vi "XDCRDefaultReader.vi"(11 "path to XML document":path=path "C:/Labview Suite/ScanningControl/Location Specific/StonyBrook/DualXDCRSettings.xml") -> (0 "Dual XDCR Settings":T1 {"XDCR Settings"."UT340 Controls"."Low Pass Filter (MHz)" min=20 step=1; "XDCR Settings"."UT340 Controls"."High Pass Filter (MHz)" min=1 max=20 step=1; "XDCR Settings"."UT340 Controls"."Pulse Width (ns)" min=2.0 max=71.75; "XDCR Settings"."UT340 Controls"."Voltage" min=100 max=250 step=2; "XDCR Settings"."UT340 Controls"."PC Gain (dB)" min=-6 max=60 step=1; "XDCR Settings"."UT340 Controls"."PE Gain (dB)" min=-6 max=60 step=1; "XDCR Settings"."JSR Complete"."JSR Trigger Settings"."PRF (Hz)" items=["100 Hz"=0.1, "200 Hz"=0.2, "400 Hz"=0.4, "600 Hz"=0.6, "800 Hz"=0.8, "1000 Hz"=1.0, "1250 Hz"=1.25, "1500 Hz"=1.5, "1750 Hz"=1.75, "2000 Hz"=2.0, "2500 Hz"=2.5, "3000 Hz"=3.0, "3500 Hz"=3.5, "4000 Hz"=4.0, "4500 Hz"=4.5, "5000 Hz"=5.0]; "XDCR Settings"."JSR Complete"."JSR Trigger Settings"."Trigger Source" items=["Internal", "External"]; "XDCR Settings"."JSR Complete"."JSR Trigger Settings"."External Trigger Limit" items=["No Limit", "5 kHz"]; "XDCR Settings"."JSR Complete"."JSR Receive Settings"."Gain (dB)" min=-13 max=66 step=1; "XDCR Settings"."JSR Complete"."JSR Receive Settings"."Low Pass Filter" items=["5 MHz"=5, "10 MHz"=10, "15 MHz"=15, "22.5 MHz"=22, "35 MHz"=35, "50 MHz"=50]; "XDCR Settings"."JSR Complete"."JSR Receive Settings"."High Pass Filter" items=["DC"=0, "1 MHz"=1000, "2.5 MHz"=2500, "5 MHz"=5000, "7.5 MHz"=7500, "12.5 MHz"=12500]; "XDCR Settings"."JSR Complete"."JSR Receive Settings"."Receiver Mode" items=["Echo", "Through"]; "XDCR Settings"."JSR Complete"."JSR Pulse Settings"."Pulser Voltage (V)" items=["100"=100, "125"=125, "150"=150, "175"=175, "200"=200, "225"=225, "250"=250, "275"=275, "300"=300, "325"=325, "350"=350, "375"=375, "400"=400, "425"=425, "450"=450, "475"=475]; "XDCR Settings"."JSR Complete"."JSR Pulse Settings"."Pulser Impedance" items=["High z", "Low z"]; "XDCR Settings"."JSR Complete"."JSR Pulse Settings"."Pulse Energy Level" items=["0 (Minimum)", "1", "2", "3 (Maximum)"]; "XDCR Settings"."JSR Complete"."JSR Pulse Settings"."Damping" items=["331 Ohms"=331, "198 Ohms"=198, "142 Ohms"=142, "110 Ohms"=110, "92 Ohms"=92, "77 Ohms"=77, "67 Ohms"=67, "59 Ohms"=59, "52 Ohms"=52, "47 Ohms"=47, "43 Ohms"=43, "39 Ohms"=39, "37 Ohms"=37, "34 Ohms"=34, "32 Ohms"=32, "30 Ohms"=30]; "XDCR Settings"."Panametrics Settings"."FINE ATTENUATION" items=["00.0", "00.5", "01.0", "01.5", "02.0", "02.5", "03.0", "03.5", "04.0", "04.5", "05.0", "05.5", "06.0", "06.5", "07.0", "07.5", "08.0", "08.5", "09.0", "09.5", "10.0", "10.5", "11.0", "11.5", "12.0", "12.5", "13.0", "13.5", "14.0", "14.5", "15.0", "15.5"]; "XDCR Settings"."Panametrics Settings"."COARSE ATTENUATION" items=["00.0", "10.0", "20.0", "30.0", "40.0", "50.0"]; "XDCR Settings"."Panametrics Settings"."GAIN (db)" items=["26.0", "40.0", "54.0"]; "XDCR Settings"."Panametrics Settings"."PRF (KHz)" items=["XREMT", "EXBNC", "0.200", "0.500", "1.000", "2.000", "5.000", "10.00", "20.00"]; "XDCR Settings"."Panametrics Settings"."MODE" items=["P/ E", "THRU", "RPP", "EXT_PLSR"]; "XDCR Settings"."Panametrics Settings"."LP FILT (MHz)" items=["20", "50", "100", "200"]; "XDCR Settings"."Panametrics Settings"."HP FILT (KHz)" items=["1", "1000", "3000", "10000"]; "XDCR Settings"."Panametrics Settings"."DAMPING (Ohm)" items=["7", "10", "16", "20", "26", "30", "40", "50"]; "XDCR Settings"."Panametrics Settings"."ENERGY (uJ)" items=["1", "2", "4", "8", "16", "32"]; "XDCR Settings"."Daxsonics Settings"."Freq (MHz)" items=["4"=4, "5"=5, "6"=6, "8"=8, "10"=10, "12"=12, "14"=14, "15"=15, "16"=16, "17"=17, "18"=18, "20"=20, "25"=25, "30"=30, "35"=35, "40"=40, "45"=45, "50"=50]; "XDCR Settings"."Daxsonics Settings"."Voltage (V)" items=["0"=0, "5"=5, "10"=10, "15"=15, "20"=20, "25"=25, "30"=30, "35"=35, "40"=40, "45"=45, "50"=50, "55"=55, "60"=60, "65"=65, "70"=70, "75"=75, "80"=80, "85"=85, "90"=90, "95"=95, "100"=100, "110"=110, "120"=120, "130"=130, "140"=140, "150"=150, "160"=160, "170"=170, "180"=180, "190"=190]; "XDCR Settings"."Daxsonics Settings"."Gain (dB)" items=["22"=22, "25"=25, "28"=28, "31"=31, "34"=34, "37"=37, "40"=40, "43"=43, "46"=46, "49"=49, "52"=52, "55"=55, "58"=58, "61"=61, "64"=64, "67"=67]; "XDCR Settings"."Digitizer Settings"."Additional dig delay (ms)" format="%.2f"; "XDCR Settings"."Digitizer Settings"."Time scale per Div" items=["100 ns"=0.1, "200 ns"=0.2, "500 ns"=0.5, "1 micros"=1.0, "2 micros"=2.0, "5 micros"=5.0, "10 micros"=10.0, "20 micros"=20.0, "50 micros"=50.0, "100 micros"=100.0, "200 micros"=200.0, "500 micros"=500.0, "1 ms"=1000.0, "2 ms"=2000.0, "5 ms"=5000.0, "10 ms"=10000.0, "20 ms"=20000.0, "50 ms"=50000.0, "100 ms"=100000.0, "200 ms"=200000.0]; "XDCR Settings"."Digitizer Settings"."RF data Sampling"."rf points per line" min=1; "XDCR Settings"."Digitizer Settings"."RF data Sampling"."Ref Delay (ms)" format="%.2f"; "XDCR Settings"."Digitizer Settings"."RF data Sampling"."Sampling Rate" items=["10 MS/s"=10.0, "20 MS/s"=20.0, "25 MS/s"=25.0, "50 MS/s"=50.0, "100 MS/s"=100.0, "200 MS/s"=200.0, "250 MS/s"=250.0, "400 MS/s"=400.0, "500 MS/s"=500.0, "1 GS/s"=1000.0]})   [LabVIEW 2022 SP3]
uses:
  Dual XDCR Complete Settings.ctl
  XDCRSettings.ctl
  Pulsers/Daxsonics/-DaxSubroutines/Dax_Control_Cluster.ctl
  Pulsers/Panametrics/Pana5900.ctl
  Pulsers/JSR/Controls/JSR Complete.ctl
  Pulsers/JSR/Controls/JSR Pulse.ctl
  Pulsers/JSR/Controls/Damping.ctl
  Pulsers/JSR/Controls/Energy.ctl
  Pulsers/JSR/Controls/Z.ctl
  Pulsers/JSR/Controls/Volt.ctl
  Pulsers/JSR/Controls/JSR Recieve.ctl
  Pulsers/JSR/Controls/Mode.ctl
  Pulsers/JSR/Controls/HPF.ctl
  Pulsers/JSR/Controls/LPF.ctl
  Pulsers/JSR/Controls/Gain.ctl
  Pulsers/JSR/Controls/JSR Trigger.ctl
  Pulsers/JSR/Controls/Trig Limit.ctl
  Pulsers/JSR/Controls/Trig Source.ctl
  Pulsers/JSR/Controls/PRF.ctl
  Pulsers/UTEX/Controls/UTEX Controls.ctl
  <vilib>/Utility/xml.llb/Read From XML File(string).vi
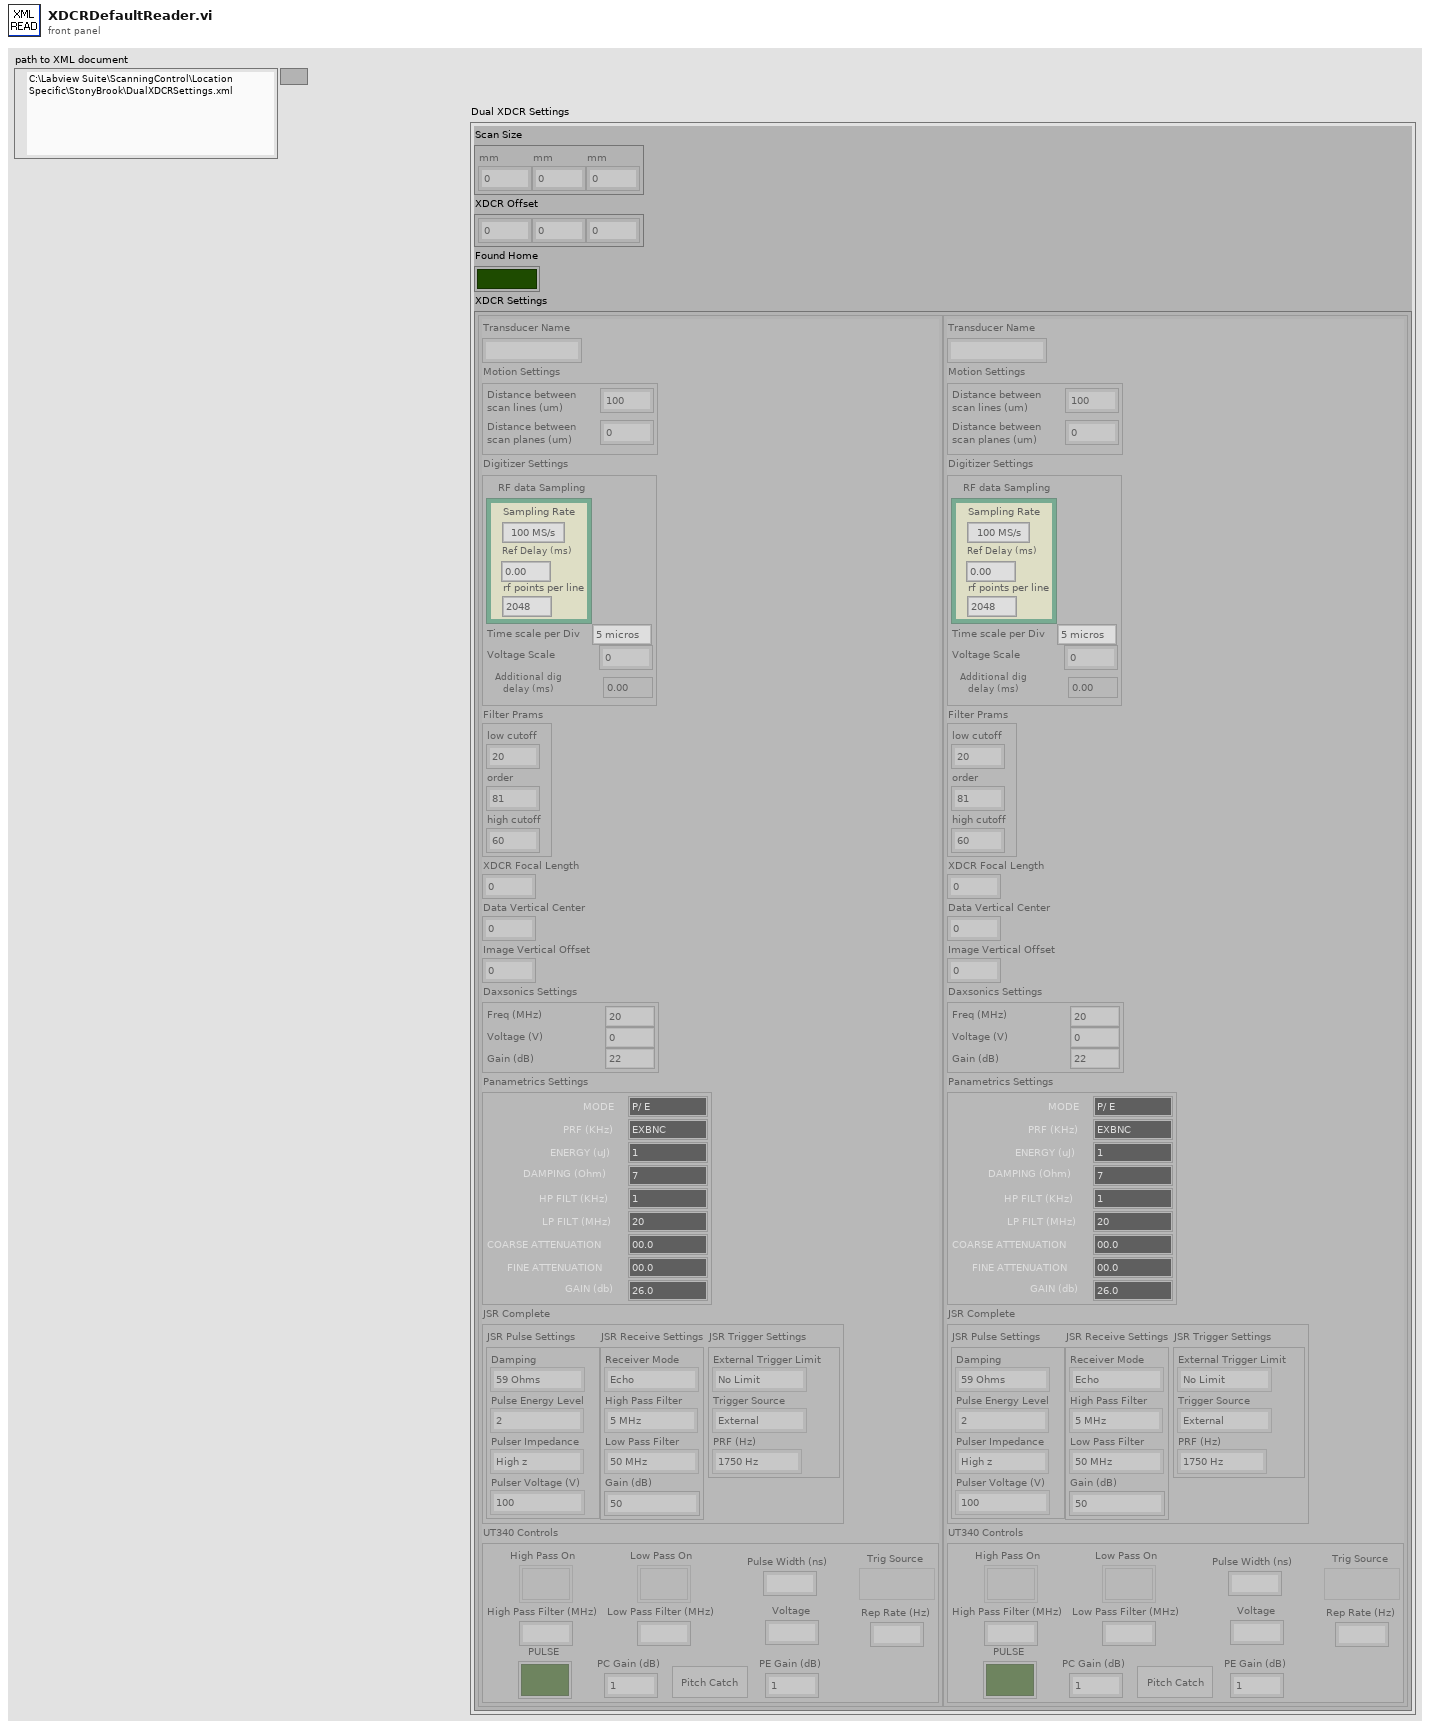
[diagram p1: front panel]
types:
  T1 = typedef "Dual XDCR Complete Settings.ctl" = cluster{"Scan Size":dbl[], "XDCR Offset":dbl[], "Found Home":bool, "XDCR Settings":T2[]}
  T2 = typedef "XDCRSettings.ctl" = cluster{"Transducer Name":string, "Motion Settings":cluster{"Distance between\nscan lines (um)":sgl, "Distance between\nscan planes (um)":sgl}, "Digitizer Settings":cluster{"RF data Sampling":cluster{"Sampling Rate":dbl, "Ref Delay (ms)":dbl, "rf points per line":i32}, "Time scale per Div":dbl, "Voltage Scale":dbl, "Additional dig delay (ms)":dbl}, "Filter Prams":cluster{"low cutoff":i32, "order":i32, "high cutoff":i32}, "XDCR Focal Length":dbl, "Data Vertical Center":dbl, "Image Vertical Offset":dbl, "Daxsonics Settings":T3, "Panametrics Settings":T4, "JSR Complete":T5, "UT340 Controls":T20}
  T3 = typedef "Dax_Control_Cluster.ctl" = cluster{"Freq (MHz) ":u16, "Voltage (V)":u16, "Gain (dB)":u16}
  T4 = typedef "Pana5900.ctl" = cluster{"ENERGY (uJ)":u16, "DAMPING (Ohm)":u16, "HP FILT (KHz) ":u16, "LP FILT (MHz)":u16, "MODE":u16, "PRF (KHz)":u16, "GAIN (db)":u16, "COARSE ATTENUATION":u16, "FINE ATTENUATION":u16}
  T5 = typedef "JSR Complete.ctl" = cluster{"JSR Pulse Settings":T6, "JSR Receive Settings":T11, "JSR Trigger Settings":T16}
  T6 = typedef "JSR Pulse.ctl" = cluster{"Damping":T7, "Pulse Energy Level":T8, "Pulser Impedance":T9, "Pulser Voltage (V)":T10}
  T7 = typedef "Damping.ctl" = i16
  T8 = typedef "Energy.ctl" = u16
  T9 = typedef "Z.ctl" = u16
  T10 = typedef "Volt.ctl" = i16
  T11 = typedef "JSR Recieve.ctl" = cluster{"Receiver Mode":T12, "High Pass Filter":T13, "Low Pass Filter":T14, "Gain (dB)":T15}
  T12 = typedef "Mode.ctl" = i8
  T13 = typedef "HPF.ctl" = u16
  T14 = typedef "LPF.ctl" = u16
  T15 = typedef "Gain.ctl" = i8
  T16 = typedef "JSR Trigger.ctl" = cluster{"External Trigger Limit":T17, "Trigger Source":T18, "PRF (Hz)":T19}
  T17 = typedef "Trig Limit.ctl" = i8
  T18 = typedef "Trig Source.ctl" = i8
  T19 = typedef "PRF.ctl" = dbl
  T20 = typedef "UTEX Controls.ctl" = cluster{"High Pass On":bool, "High Pass Filter (MHz)":i16, "Low Pass On":bool, "Low Pass Filter (MHz)":i16, "PE Gain (dB)":i16, "Voltage":i16, "Pulse Width (ns)":dbl, "Mode":bool, "PC Gain (dB)":i16, "Trig Source":bool, "Rep Rate (Hz)":i16, "PULSE":bool}
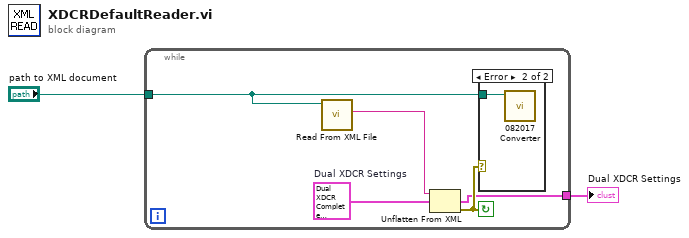
[diagram p0: block diagram]
diagram:
  n1 = while {
    tunnel: "path to XML document" -> [w7]
    tunnel: [w3] -> w1
    stop <- w4 continue-if-true
    w5 = T1 {"Scan Size"=[20.0, 20.0, 12.5], "XDCR Offset"=[0.0, -35.7, 14.5], "Found Home"=FALSE, "XDCR Settings"=[]}  # Dual XDCR Settings
    n2 = call-poly <vilib>:"Read From XML File.vi"("XML File Path"=w7) -> ("XML Elements"=w6:string)  [unwired: 8 in, 2 out]
    n3 = Unflatten From XML(xml string=w6, type=w5) -> (value=w3:T1, error out=w4:errorcluster)  [unwired: 1 in]
    n4 = case shown="Error" w4 {
      tunnel: w7 -> [_ w8]
      frame No Error {
      }
      frame Error {
        n5 = call "082017 Converter.vi"("path to XML document"=w8) -> ()  [unwired: 10 in, 1 out]
      }
    }
  }
  "Dual XDCR Settings" <- w1
